vi "Day 6 task 1.vi"() -> ()   [LabVIEW 2022 SP3]
panel:
  out "Numeric":i32
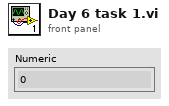
[diagram p1: front panel]
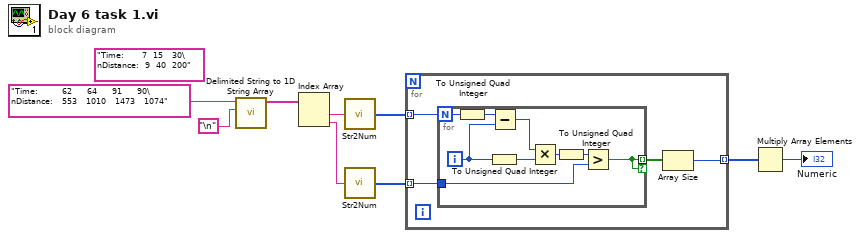
[diagram p0: block diagram]
diagram:
  (unwired) "Time:      7  15   30\nDistance:  9  40  200"
  n1 = call <vilib>:"Delimited String to 1D String Array.vi"("delimiter"="\n", "delimited string"="Time:        62     64     91     90\nDistance:   553   1010   1473   1074") -> ("string array"=w8:string[])  [unwired: 9 in]
  n2 = Index Array(array=w8) -> (element #1=w7:string, element #2=w6:string)  [unwired: 2 in]
  n3 = call "Str2Num.vi"("str_data"=w7) -> ("arr_values"=w5:u64[])  [unwired: 8 in]
  n4 = call "Str2Num.vi"("str_data"=w6) -> ("arr_values"=w4:u64[])  [unwired: 8 in]
  n5 = for {
    tunnel: w5 -> [w13] mode=indexing
    tunnel: w4 -> [w12] mode=indexing
    tunnel: [w10] -> w3 mode=indexing
    n6 = for {
      N: w13 -> [w22]
      tunnel: w12 -> [w18]
      tunnel: [w17] -> w11 mode=indexing if=w17
      i -> [w20]
      n7 = To Unsigned Quad Integer(1:w22) -> (0:w16:u64)
      n8 = To Unsigned Quad Integer(1:w20) -> (0:w15:u64)
      n9 = Subtract(x=w16, y=w20) -> (x-y=w21:u64)
      n10 = Multiply(x=w21, y=w15) -> (x*y=w19:u64)
      n11 = To Unsigned Quad Integer(1:w19) -> (0:w14:u64)
      n12 = Greater?(x=w14, y=w18) -> (0:w17:bool)
    }
    n13 = Array Size(array=w11) -> (size(s)=w10:i32)
  }
  n14 = Multiply Array Elements(1:w3) -> (0:→"Numeric":i32)
